vi "Scale and stream to TDMS.vi"(11 "Logging queue element in":T1={"Imaging Protocol"=enum."Functional Acquisition", "Number of Trials"=2, "Frame Size"=200, "# Averaged frames"=1, "Dwell time (us)"=0.1, "Index of Z-plane"=0, "Timelapse?"=FALSE, "Logging process is active"=TRUE, "Speed logging enabled"=FALSE, "tdms file ref"=refnum, "path"=path "D:/Microscope data/2015-July-02/150702_14_41_11/Functional imaging TDMS data files/002.tdms", "Trial Number"=2, "Expected # points acquired"=TRUE, "Manually stopped"=FALSE, "Ch0 data"=array[10032 elements], "Ch1 data"=array[10032 elements], "Ref Data"=[], "Last trial"=FALSE, "Ref Dwell time (us)"=0.20000000298023224, "# Ref Averaged frames"=1, "Ref X Length"=0, "Ref Y Length"=0, "Points acquired"={"Ch0 last trial"=6346380, "Ch1 last trial"=6346380, "All trials"=12692760}} {"Ref Dwell time (us)" format="%#.6g"; "Frame Size" items=["100X100"=100, "128X128"=128, "200X200"=200, "256X256"=256, "512X512"=512, "1024x1024"=1024, "2048x2048"=2048]; "Dwell time (us)" format="%#.6g"}) -> (0 "error out":errorcluster, 2 "Expected # points acquired":bool, 3 "Refnum out":refnum<k34>)   [LabVIEW 2017]
uses:
  <vilib>/Analysis/NI_AALBase.lvlib
  <vilib>/Analysis/baseanly.llb/Mean (DBL).vi
  Typedefs/Imaging Protocols enum.ctl
  Typedefs/Frame Size.ctl
  Typedefs/Acquired points count.ctl
  Typedefs/Logging queue element.ctl
panel:
  in  "stop":bool
  out "Loop":i32
  out "Average ms":dbl format="%_6f"
  in  "file path":path
  out "x-y":dbl format="%_6f"
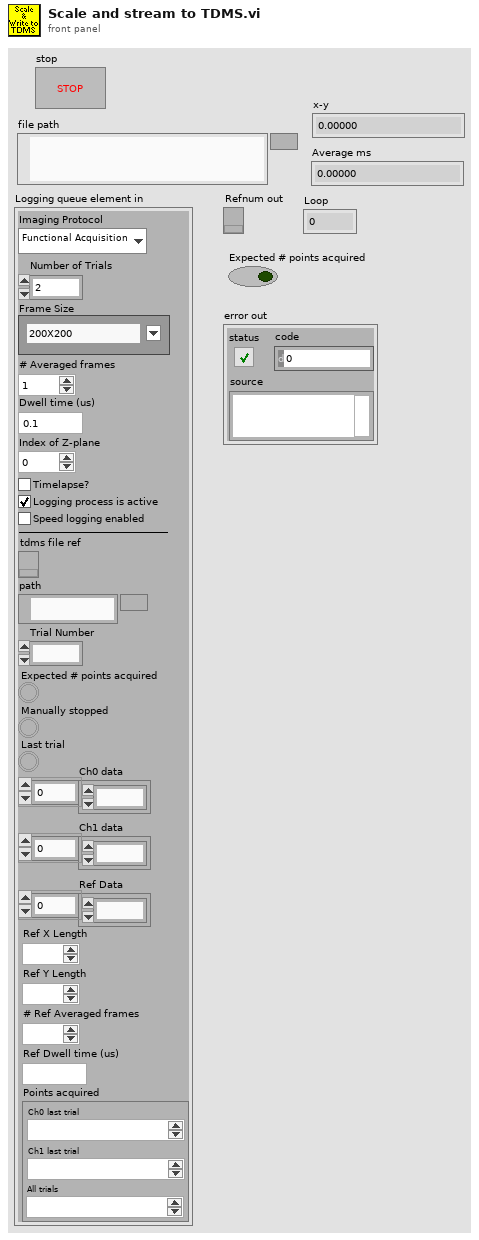
[diagram p1: front panel]
types:
  T1 = typedef "Logging queue element.ctl" = cluster{"Imaging Protocol":T2, "Number of Trials":u16, "Frame Size":T3, "# Averaged frames":u16, "Dwell time (us)":dbl, "Index of Z-plane":i32, "Timelapse?":bool, "Logging process is active":bool, "Speed logging enabled":bool, "tdms file ref":refnum<k34>, "path":path, "Trial Number":i32, "Expected # points acquired":bool, "Manually stopped":bool, "Ch0 data":u32[], "Ch1 data":u32[], "Ref Data":u32[], "Last trial":bool, "Ref Dwell time (us)":dbl, "# Ref Averaged frames":u16, "Ref X Length":u16, "Ref Y Length":u16, "Points acquired":T4}
  T2 = typedef "Imaging Protocols enum.ctl" = enum16{"AOL Z-Stack", "Motor Z Stack", "Functional Acquisition", "Single Plane Acquisition", "Volume Acquisition", "Live Imaging", "Live Plane Imaging", "Live Volume Imaging"}
  T3 = typedef "Frame Size.ctl" = u16
  T4 = typedef "Acquired points count.ctl" = cluster{"Ch0 last trial":u64, "Ch1 last trial":u64, "All trials":u64}
  T5 = enum16{"open", "open or create", "create or replace", "create", "open (read-only)"}
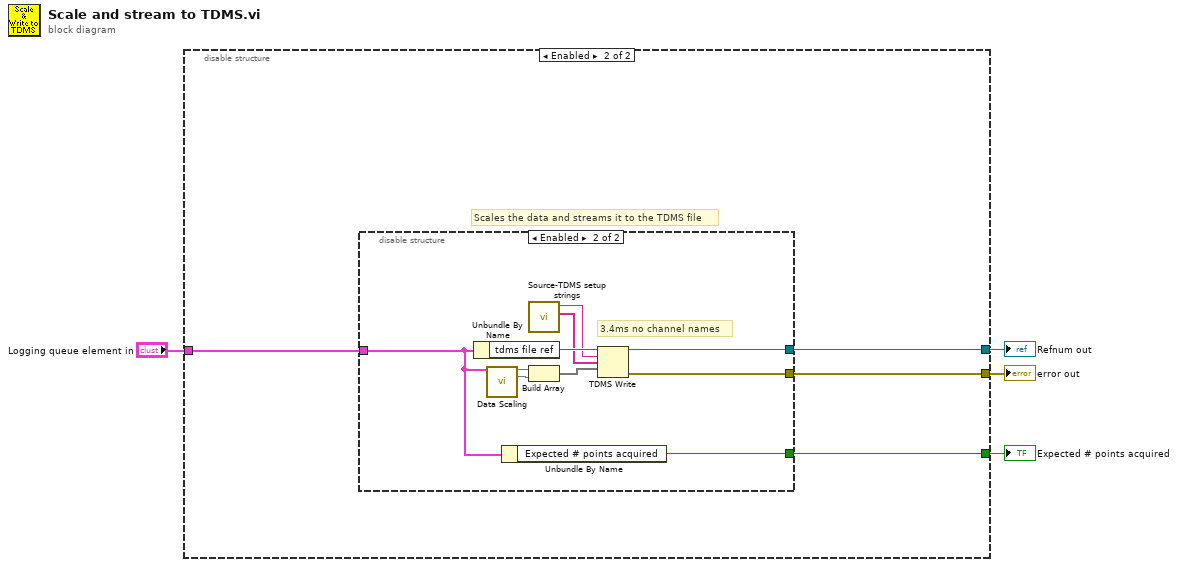
[diagram p0: block diagram]
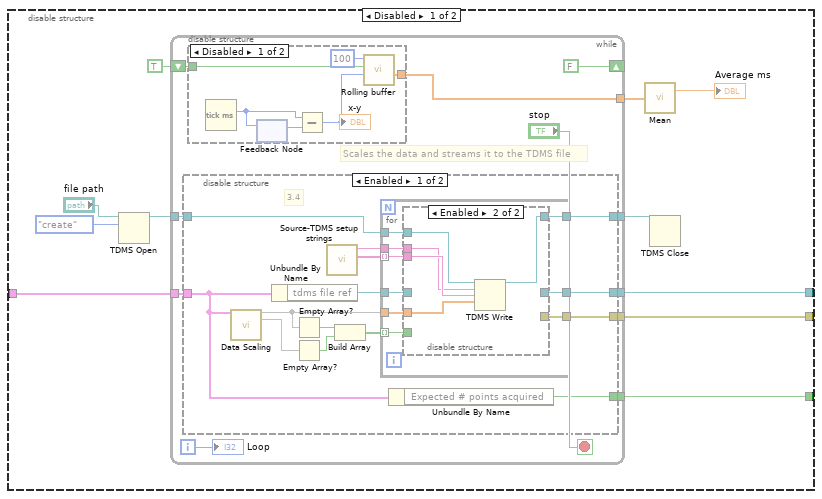
[diagram p2: hidden frame]
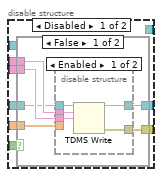
[diagram p4: hidden frame]
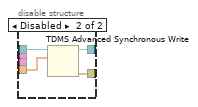
[diagram p5: hidden frame]
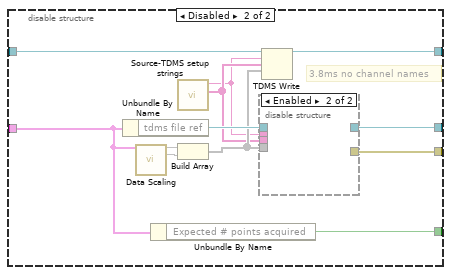
[diagram p7: hidden frame]
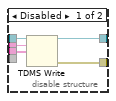
[diagram p8: hidden frame]
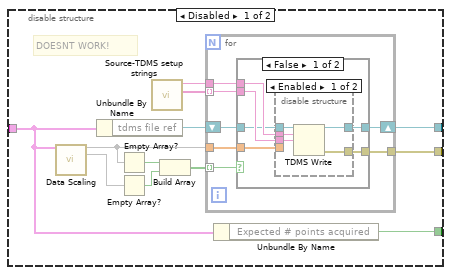
[diagram p9: hidden frame]
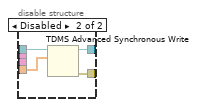
[diagram p10: hidden frame]
diagram:
  n1 = disable-structure shown="Enabled" {
    disable-tunnel: [w15 w106] -> w4
    disable-tunnel: [w14 w105] -> w3
    disable-tunnel: "Logging queue element in" -> [w13 w104]
    disable-tunnel: [w12 w103] -> w1
    frame Disabled {
      n2 = TDMS Open(10:T5."create" ("operation (0:open)"), 11:"file path") -> (3:w11:refnum<k34>)  [unwired: 5 in, 1 out]
      n3 = while {
        tunnel: [w26] -> w15
        tunnel: [w25] -> w14
        tunnel: w13 -> [w24]
        tunnel: [w23] -> w12
        tunnel: w11 -> [w21]
        tunnel: [w20] -> w10
        shift-right: [FALSE] -> _
        shift-left: TRUE -> [w19]
        tunnel: [w16] -> w5
        i -> [w17]
        stop <- "stop" stop-if-true
        # "Scales the data and streams it to the TDMS file"
        n4 = disable-structure shown="Enabled" {
          disable-tunnel: [w44 w96] -> w26
          disable-tunnel: [w43 w95] -> w25
          disable-tunnel: w24 -> [w39 w93]
          disable-tunnel: [w38 w92] -> w23
          disable-tunnel: w21 -> [w34 w89]
          disable-tunnel: [w33 w88] -> w20
          frame Enabled {
            # "3.4"
            n5 = call "Data Scaling.vi"("Logging queue element in"=w39) -> (4:w41, 6:w40)  [unwired: 11 in, 2 out]
            n6 = Unbundle By Name(w39) -> ("tdms file ref"=w42:refnum<k34>)
            n7 = Empty Array?(array=w41) -> (empty?=w37:bool)
            n8 = Empty Array?(array=w40) -> (empty?=w36:bool)
            n9 = call "Source-TDMS setup strings.vi"() -> ("Functional imaging TDMS channel names array"=w45:string[], "TDMS group name"=w46:string)  [unwired: 10 in]
            n10 = Build Array(w37, w36) -> (w35:bool[])
            n11 = for {
              tunnel: w46 -> [w55]
              tunnel: w45 -> [w54] mode=indexing
              tunnel: [w53] -> w44
              tunnel: [w52] -> w43
              tunnel: w42 -> [w51]
              tunnel: w41 -> [w50]
              tunnel: w35 -> [w49] mode=indexing
              tunnel: w34 -> [w48]
              tunnel: [w47] -> w33
              n12 = disable-structure shown="Enabled" {
                disable-tunnel: w55 -> [w62 w80]
                disable-tunnel: w54 -> [w61 w81]
                disable-tunnel: [w60 _] -> w53
                disable-tunnel: [w59 _] -> w52
                disable-tunnel: w51 -> [w58 _]
                disable-tunnel: w50 -> [w57 w82]
                disable-tunnel: w49 -> [w56 _]
                disable-tunnel: w48 -> [_ w84]
                disable-tunnel: [_ w83] -> w47
                frame Disabled {
                  n13 = case shown="False" w56 {
                    tunnel: w62 -> [w68 _]
                    tunnel: w61 -> [w67 _]
                    tunnel: [w66 w79] -> w60
                    tunnel: [w65 _] -> w59
                    tunnel: w58 -> [w64 w79]
                    tunnel: w57 -> [w63 _]
                    frame False {
                      n14 = disable-structure shown="Enabled" {
                        disable-tunnel: w68 -> [w74 _]
                        disable-tunnel: w67 -> [w73 _]
                        disable-tunnel: [w72 w77] -> w66
                        disable-tunnel: [w71 w76] -> w65
                        disable-tunnel: w64 -> [w70 w78]
                        disable-tunnel: w63 -> [w69 w75]
                        frame Enabled {
                          n15 = TDMS Write(0:w70, 5:w74, 7:w73, 9:w69) -> (4:w72:refnum<k34>, 15:w71:errorcluster)  [unwired: 2 in, 2 out]
                        }
                        frame Disabled {
                          n16 = TDMS Advanced Synchronous Write(10:w75, 11:w78) -> (0:w76:errorcluster, 3:w77:refnum<k34>)  [unwired: 1 in]
                        }
                      }
                    }
                    frame True {
                    }
                  }
                }
                frame Enabled {
                  n17 = TDMS Write(0:w84, 5:w80, 7:w81, 9:w82) -> (4:w83:refnum<k34>)  [unwired: 2 in, 3 out]
                }
              }
            }
            n18 = Unbundle By Name(w39) -> ("Expected # points acquired"=w38:bool)
          }
          frame Disabled {
            # "3.8ms no channel names"
            n19 = Unbundle By Name(w93) -> ("tdms file ref"=w94:refnum<k34>)
            n20 = call "Data Scaling.vi"("Logging queue element in"=w93) -> (4:w90, 6:w91)  [unwired: 11 in, 2 out]
            n21 = Unbundle By Name(w93) -> ("Expected # points acquired"=w92:bool)
            n22 = call "Source-TDMS setup strings.vi"() -> ("Functional imaging TDMS channel names array"=w86:string[], "TDMS group name"=w85:string)  [unwired: 10 in]
            n23 = Build Array(w90, w91) -> (w87:void[])
            n24 = disable-structure shown="Enabled" {
              disable-tunnel: w85 -> [w102 _]
              disable-tunnel: w86 -> [w101 _]
              disable-tunnel: [w100 _] -> w96
              disable-tunnel: [w99 _] -> w95
              disable-tunnel: w94 -> [w98 _]
              disable-tunnel: w87 -> [w97 _]
              frame Disabled {
                n25 = TDMS Write(0:w98, 5:w102, 7:w101, 9:w97) -> (4:w100:refnum<k34>, 15:w99:errorcluster)  [unwired: 2 in, 2 out]
              }
              frame Enabled {
              }
            }
            n26 = TDMS Write(0:w89, 5:w85, 7:w86, 9:w87) -> (4:w88:refnum<k34>)  [unwired: 2 in, 3 out]
          }
        }
        n27 = disable-structure shown="Disabled" {
          disable-tunnel: w19 -> [w31 _]
          disable-tunnel: [w27 _] -> w16
          frame Disabled {
            n28 = Tick Count (ms)() -> (millisecond timer value=w29:u32)
            n29 = feedback #1() -> (w32:u32)  [unwired: 1 in]
            n30 = feedback-in #1(w29) -> ()
            n31 = Subtract(x=w29, y=w32) -> (x-y=w28:u32)
            "x-y" <- w28
            n32 = call "Rolling buffer.vi"("Value in"=w28, "Reset buffer"=w31, "Buffer length (points)"=100) -> ("Rolling buffer"=w27:dbl[])  [unwired: 8 in]
          }
          frame Enabled {
          }
        }
        "Loop" <- w17
      }
      n33 = call-poly <vilib>:"Mean.vi"("X"=w5) -> ("mean"=→"Average ms":dbl)  [unwired: 1 out]
      n34 = TDMS Close(11:w10) -> ()  [unwired: 1 in, 2 out]
    }
    frame Enabled {
      # "Scales the data and streams it to the TDMS file"
      n35 = disable-structure shown="Enabled" {
        disable-tunnel: [w107 w152] -> w106
        disable-tunnel: [w116 w151] -> w105
        disable-tunnel: w104 -> [w112 w149]
        disable-tunnel: [w111 w148] -> w103
        frame Disabled {
          # "DOESNT WORK!"
          n36 = call "Data Scaling.vi"("Logging queue element in"=w112) -> (4:w114, 6:w113)  [unwired: 11 in, 2 out]
          n37 = Unbundle By Name(w112) -> ("tdms file ref"=w115:refnum<k34>)
          n38 = Empty Array?(array=w114) -> (empty?=w110:bool)
          n39 = Empty Array?(array=w113) -> (empty?=w109:bool)
          n40 = call "Source-TDMS setup strings.vi"() -> ("Functional imaging TDMS channel names array"=w117:string[], "TDMS group name"=w118:string)  [unwired: 10 in]
          n41 = Build Array(w110, w109) -> (w108:bool[])
          n42 = for {
            tunnel: w118 -> [w125]
            tunnel: w117 -> [w124] mode=indexing
            tunnel: [w123] -> w116
            tunnel: w114 -> [w121]
            tunnel: w108 -> [w120] mode=indexing
            shift-right: [w119] -> w107
            shift-left: w115 -> [w122]
            n43 = case shown="False" w120 {
              tunnel: w125 -> [w131 _]
              tunnel: w124 -> [w130 _]
              tunnel: [w129 w142] -> w119
              tunnel: [w128 _] -> w123
              tunnel: w122 -> [w127 w142]
              tunnel: w121 -> [w126 _]
              frame False {
                n44 = disable-structure shown="Enabled" {
                  disable-tunnel: w131 -> [w137 _]
                  disable-tunnel: w130 -> [w136 _]
                  disable-tunnel: [w135 w140] -> w129
                  disable-tunnel: [w134 w139] -> w128
                  disable-tunnel: w127 -> [w133 w141]
                  disable-tunnel: w126 -> [w132 w138]
                  frame Enabled {
                    n45 = TDMS Write(0:w133, 5:w137, 7:w136, 9:w132) -> (4:w135:refnum<k34>, 15:w134:errorcluster)  [unwired: 2 in, 2 out]
                  }
                  frame Disabled {
                    n46 = TDMS Advanced Synchronous Write(10:w138, 11:w141) -> (0:w139:errorcluster, 3:w140:refnum<k34>)  [unwired: 1 in]
                  }
                }
              }
              frame True {
              }
            }
          }
          n47 = Unbundle By Name(w112) -> ("Expected # points acquired"=w111:bool)
        }
        frame Enabled {
          # "3.4ms no channel names"
          n48 = Unbundle By Name(w149) -> ("tdms file ref"=w150:refnum<k34>)
          n49 = call "Data Scaling.vi"("Logging queue element in"=w149) -> (4:w146, 6:w147)  [unwired: 11 in, 2 out]
          n50 = Unbundle By Name(w149) -> ("Expected # points acquired"=w148:bool)
          n51 = call "Source-TDMS setup strings.vi"() -> ("Functional imaging TDMS channel names array"=w144:string[], "TDMS group name"=w143:string)  [unwired: 10 in]
          n52 = Build Array(w146, w147) -> (w145:void[])
          n53 = TDMS Write(0:w150, 5:w143, 7:w144, 9:w145) -> (4:w152:refnum<k34>, 15:w151:errorcluster)  [unwired: 2 in, 2 out]
        }
      }
    }
  }
  "Expected # points acquired" <- w1
  "Refnum out" <- w4
  "error out" <- w3
